vi "JsonFile_GetAttribute(DBL).vi"(8 "error in (no error)":errorcluster, 9 "Default Value":dbl, 10 "Attribute":string, 11 "Json":path) -> (0 "error out":errorcluster, 1 "Found?":bool, 2 "Value":dbl, 3 "Json":path)   [LabVIEW 2019, in "lv-apt-json-file.lvlib"]
uses:
  <userlib>/_lvAPT/lv-apt-json-file/lv-apt-json-file.lvlib
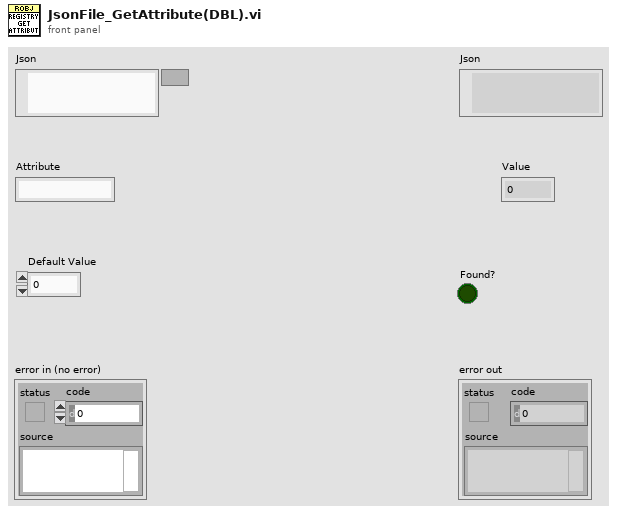
[diagram p1: front panel]
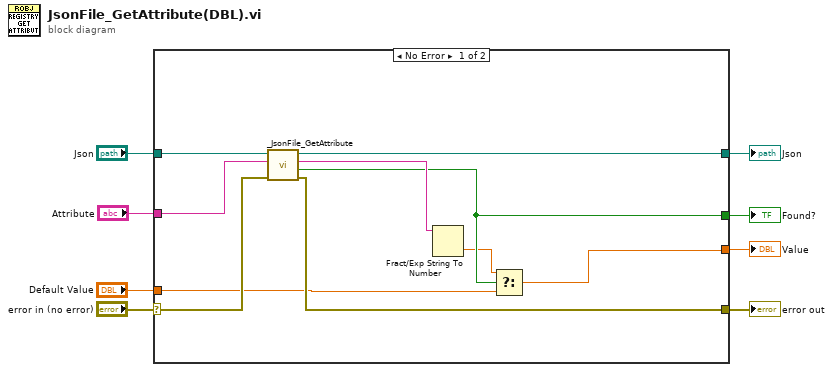
[diagram p0: block diagram]
diagram:
  n1 = case shown="No Error" "error in (no error)" {
    selector: "error in (no error)" -> [w16 w20]
    tunnel: "Json" -> [w17 w19]
    tunnel: "Attribute" -> [w18 _]
    tunnel: [w15 w19] -> w6
    tunnel: [w14 w20] -> w4
    tunnel: [w12 _] -> w3
    tunnel: [w9 _] -> w2
    tunnel: "Default Value" -> [w11 _]
    frame No Error {
      n2 = call <userlib>:"_JsonFile_GetAttribute.vi"("error in (no error)"=w16, "Attribute"=w18, "Json"=w17) -> ("error out"=w14:errorcluster, "Found?"=w12:bool, "String"=w13:string, "Json (dup)"=w15:path)  [unwired: 5 in]
      n3 = Fract/Exp String To Number(string=w13) -> (number=w10:dbl)  [unwired: 3 in, 1 out]
      n4 = Select(t=w10, s=w12, f=w11) -> (s? t:f=w9:dbl)
    }
    frame Error {
    }
  }
  "error out" <- w4
  "Json" <- w6
  "Value" <- w2
  "Found?" <- w3
